vi "startPlayback.vi"(8 "error in (no error)":errorcluster, 11 "Player in":refnum<class "Player.lvclass">) -> (0 "error out":errorcluster, 2 "Song":string, 3 "Player out":refnum<class "Player.lvclass">)   [LabVIEW 2017, in "Player.lvclass"]
uses:
  Player.lvclass
  Player.lvclass/Player.ctl
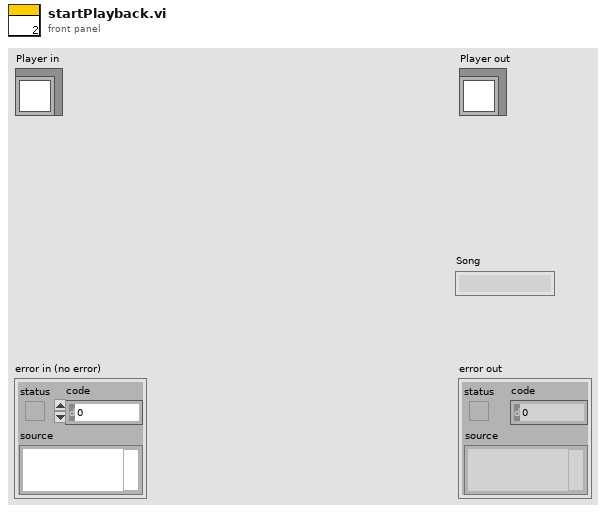
[diagram p1: front panel]
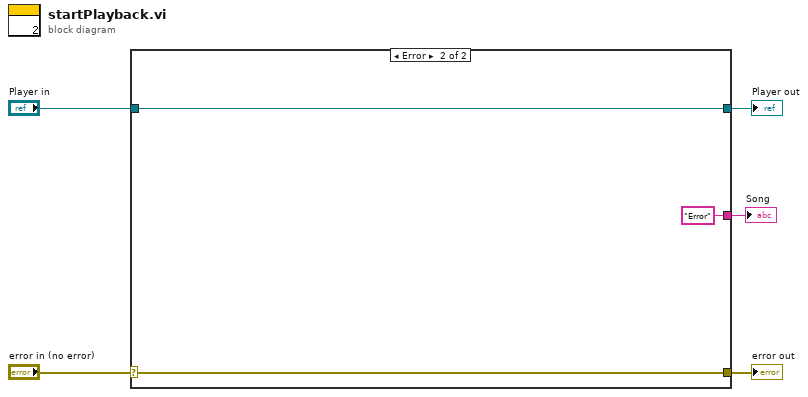
[diagram p0: block diagram]
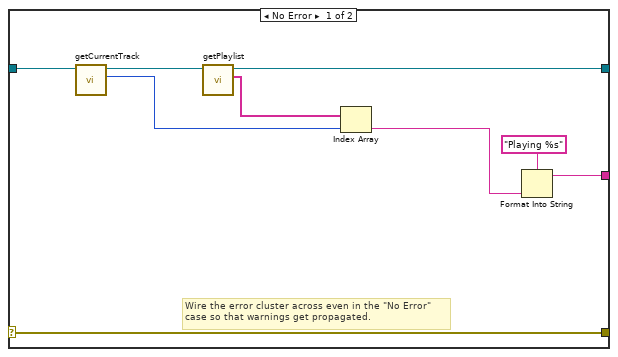
[diagram p2: hidden frame]
diagram:
  n1 = case shown="Error" "error in (no error)" {
    selector: "error in (no error)" -> [w13 w17]
    tunnel: [w13 w17] -> w4
    tunnel: [w11 w16] -> w2
    tunnel: "Player in" -> [w14 w16]
    tunnel: [w7 "Error"] -> w1
    frame No Error {
      # "Wire the error cluster across even in the \"No Error\"\ncase so that warnings get propagated."
      n2 = call "getCurrentTrack.vi"("Player in"=w14) -> ("currentTrack"=w9:u32, "Player out"=w12:refnum<class "Player.lvclass">)  [unwired: 8 in, 1 out]
      n3 = call "getPlaylist.vi"("Player in"=w12) -> ("Playlist"=w10:string[], "Player out"=w11:refnum<class "Player.lvclass">)  [unwired: 8 in, 1 out]
      n4 = Index Array(array=w10, index=w9) -> (element=w6:string)
      n5 = Format Into String(format string="Playing %s", w6) -> (resulting string=w7:string)  [unwired: 2 in, 1 out]
    }
    frame Error {
    }
  }
  "error out" <- w4
  "Player out" <- w2
  "Song" <- w1
